vi "Sim_Elevator.vi"(9 "StartPosInches":dbl, 10 "Motor2 Dmd":dbl=6.0, 11 "Motor1 Dmd":dbl) -> (1 "HighLimitSwitch":bool, 2 "Low Limit Switch":bool, 3 "ElevHeightInch":dbl, 4 "Voltage":dbl)   [LabVIEW 2023]
uses:
  <vilib>/Rock Robotics/WPI/ThirdParty/JAS_Junk/TrajLib/Enum/DCMOTOR_TYPES_ENUM.ctl
  <vilib>/Rock Robotics/WPI/ThirdParty/JAS_Junk/TrajLib/BatterySim_CalculateLoadedBatteryVoltage.vi
  <vilib>/Rock Robotics/WPI/ThirdParty/JAS_Junk/TrajLib/Trajectory_Library.lvlib
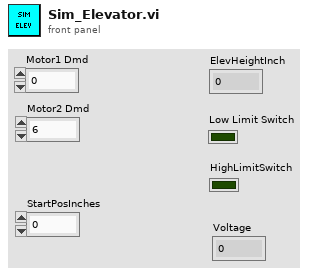
[diagram p1: front panel]
types:
  T1 = typedef "Trajectory_Library.lvlib/DCMOTOR_TYPES_ENUM.ctl" = enum16{"CIM", "AndyMark 9015", "Andy Mark RS 775 125", "Bag", "BaneBots RS 550", "BaneBots RS 775", "Falcon 500", "Mini CIM", "NEO", "NEO 550", "Romi BuiltIn", "Vex 775 Pro", "Snow Blower AM 2235A", "Bosch Seat AM 3493", "Falcon 500 FOC", "Kraken X60", "Kraken X60 FOC", "NEO Vortex"}
  T2 = typedef "Trajectory_Library.lvlib/LINEAR_SYSTEM_ID_ELEVATOR_MODEL.CTL" = cluster{"DCMOTOR_TYPES":T1, "Num Motors":i32, "WinchRadias_Meters":dbl, "mass_Kg":dbl, "Gearing":dbl}
  T3 = typedef "Trajectory_Library.lvlib/ELEVATOR_SIM_SIMULATION_PARAMS.ctl" = cluster{"MinHeight_Meters":dbl, "MaxHeight_Meters":dbl, "Measurment StdDev":dbl, "SimulateGravity":bool}
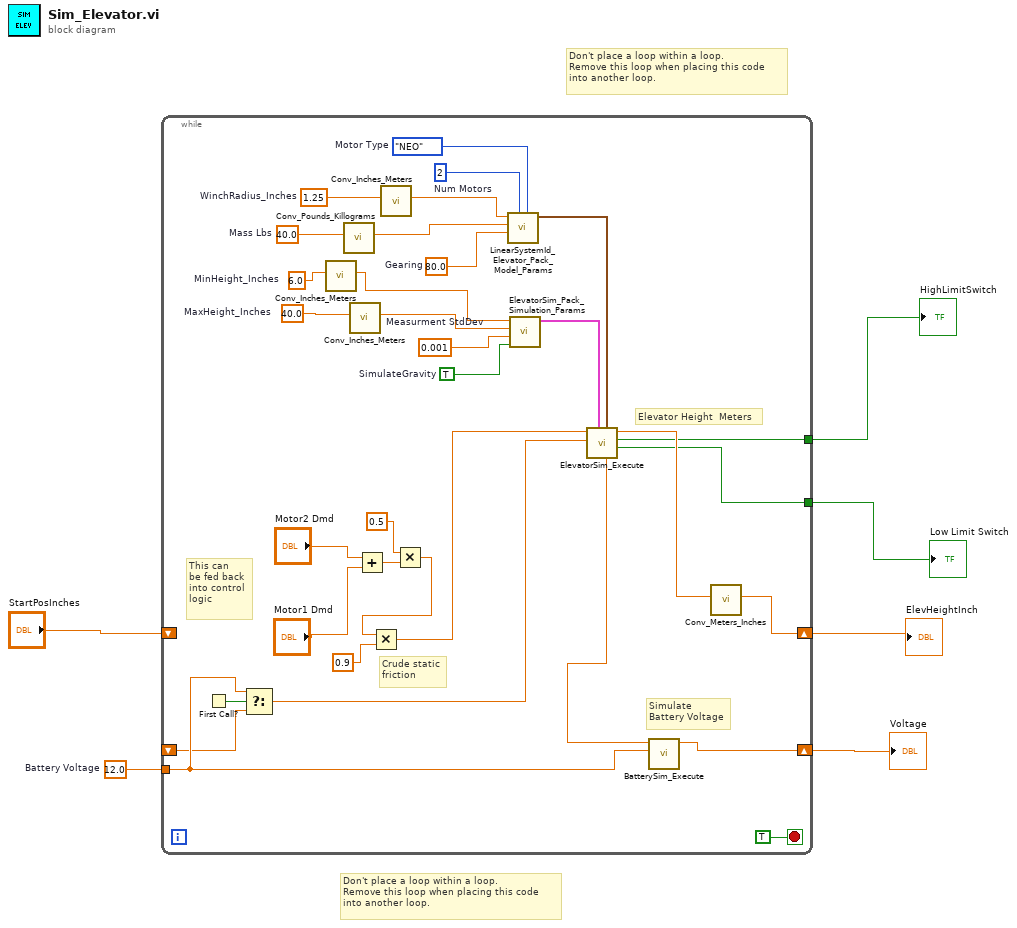
[diagram p0: block diagram]
diagram:
  w6 = 12.0  # Battery Voltage
  # "Don't place a loop within a loop. \nRemove this loop when placing this code\ninto another loop."
  # "Don't place a loop within a loop. \nRemove this loop when placing this code\ninto another loop."
  n1 = while {
    shift-right: [w39] -> w1
    shift-left: _ -> [w35]
    shift-right: [w18] -> w5
    shift-left: "StartPosInches" -> [_]
    tunnel: w6 -> [w36]
    tunnel: [w15] -> w4
    tunnel: [w14] -> w3
    stop <- TRUE stop-if-true
    w23 = 6.0  # MinHeight_Inches
    w22 = 40.0  # MaxHeight_Inches
    w30 = 0.001  # Measurment StdDev
    w31 = TRUE  # SimulateGravity
    w26 = 1.25  # WinchRadius_Inches
    w32 = 80.0  # Gearing
    w25 = 40.0  # Mass Lbs
    w33 = 2  # Num Motors
    w34 = DCMOTOR_TYPES_ENUM."NEO"  # Motor Type
    # "Elevator Height  Meters"
    # "Crude static\nfriction"
    # "This can\nbe fed back\ninto control\nlogic"
    # "Simulate\nBattery Voltage"
    n2 = First Call?() -> (First Call?: T/F=w37:bool)
    n3 = Select(t=w36, s=w37, f=w35) -> (s? t:f=w16:dbl)
    n4 = call <vilib>:"Conv_Inches_Meters.vi"("INCH"=w23) -> ("Meters"=w21:dbl)  [unwired: 10 in]
    n5 = call <vilib>:"Conv_Pounds_Killograms.vi"("Pounds"=w25) -> ("Killograms"=w24:dbl)  [unwired: 10 in]
    n6 = call <vilib>:"Conv_Inches_Meters.vi"("INCH"=w22) -> ("Meters"=w20:dbl)  [unwired: 10 in]
    n7 = Add(x="Motor2 Dmd", y="Motor1 Dmd") -> (x+y=w10:dbl)
    n8 = call <vilib>:"Conv_Inches_Meters.vi"("INCH"=w26) -> ("Meters"=w27:dbl)  [unwired: 10 in]
    n9 = Multiply(x=0.5, y=w10) -> (x*y=w8:dbl)
    n10 = Multiply(x=w8, y=0.9) -> (x*y=w17:dbl)
    n11 = call <vilib>:"LinearSystemId_Elevator_Pack_Model_Params.vi"("DCMOTOR_TYPES"=w34, "Num Motors"=w33, "Gearing"=w32, "mass_Kg"=w24, "WinchRadius_Meters"=w27) -> ("Elevator_Model _Params"=w29:T2)  [unwired: 6 in]
    n12 = call <vilib>:"ElevatorSim_Pack_Simulation_Params.vi"("SimulateGravity"=w31, "Measurment StdDev"=w30, "MaxHeight_Meters"=w20, "MinHeight_Meters"=w21) -> ("ElevatorSim_Simulation _Params"=w28:T3)  [unwired: 7 in]
    n13 = call <vilib>:"ElevatorSim_Execute.vi"("LinearSystemID_Elevator_Model _Params"=w29, "ElevatorSim_Simulation _Params"=w28, "Battery Volts"=w16, "Motor Dmd"=w17) -> ("AtLowLimit"=w14:bool, "At HIgh LImit"=w15:bool, "ElevatorHeight_Meters"=w19:dbl, "Motor Current"=w13:dbl)  [unwired: 2 in, 2 out]
    n14 = call <vilib>:"BatterySim_Execute.vi"("Nominal Battery Voltage"=w36, "Current"=w13) -> ("Voltage"=w39:dbl)  [unwired: 9 in]
    n15 = call <vilib>:"Conv_Meters_Inches.vi"("Meters"=w19) -> ("Inches"=w18:dbl)  [unwired: 10 in]
  }
  "ElevHeightInch" <- w5
  "Low Limit Switch" <- w3
  "HighLimitSwitch" <- w4
  "Voltage" <- w1
